vi "CLIENT_read_config_files_to_fgv.vi"(8 "error_in":errorcluster, 11 "all_config_info_in":T1={"main_ini_file"={"SQL Driver"="", "SQL Server"="", "SQL Database"="", "SQL UID"="", "Reference table"="", "Reference history"="", "Archivisation CFG table"="", "Archivisation CFG history"="", "User table"="", "User history"="", "logout timeout [ms]"=0, "records per page"=0, "default language"="", "REF CHG connection IP"="", "REF CHG remote port"=0, "REF CHG local port"=0, "SCANNER COM port"=0, "SCANNER Baud rate"=0, "SCANNER Data bits"=0, "SCANNER Pairity"=enum."None", "SCANNER Stop bits"=10, "SCANNER Flow control"=0, "SCANNER Termination char"=0}, "SQL Password"="", "queue_refnums"={"SQL_EDITOR_queue"=refnum, "SCANNER_queue"=refnum, "SCANNER_data"=refnum, "CLIENT_REF_CHG_queue"=refnum}} {"main_ini_file"."SCANNER Flow control" items=["None"=0, "XON/XOFF"=1, "RTS/CTS"=2, "DTR/DSR"=4]; "main_ini_file"."SCANNER Stop bits" items=["1.0"=10, "1.5"=15, "2.0"=20]}) -> (0 "error_out":errorcluster, 3 "all_config_info_out":T1={"main_ini_file"={"SQL Driver"="", "SQL Server"="", "SQL Database"="", "SQL UID"="", "Reference table"="", "Reference history"="", "Archivisation CFG table"="", "Archivisation CFG history"="", "User table"="", "User history"="", "logout timeout [ms]"=0, "records per page"=0, "default language"="", "REF CHG connection IP"="", "REF CHG remote port"=0, "REF CHG local port"=0, "SCANNER COM port"=0, "SCANNER Baud rate"=0, "SCANNER Data bits"=0, "SCANNER Pairity"=enum."None", "SCANNER Stop bits"=10, "SCANNER Flow control"=0, "SCANNER Termination char"=0}, "SQL Password"="", "queue_refnums"={"SQL_EDITOR_queue"=refnum, "SCANNER_queue"=refnum, "SCANNER_data"=refnum, "CLIENT_REF_CHG_queue"=refnum}} {"main_ini_file"."SCANNER Flow control" items=["None"=0, "XON/XOFF"=1, "RTS/CTS"=2, "DTR/DSR"=4]; "main_ini_file"."SCANNER Stop bits" items=["1.0"=10, "1.5"=15, "2.0"=20]})   [LabVIEW 2019]
uses:
  typedef/CLIENT_all_config_info.ctl
  typedef/CLIENT_main_ini_file.ctl
  queues/typedef/CLIENT_queue_refnums.ctl
  queues/typedef/SQL_EDITOR_queue_element.ctl
  MAIN/SQL_EDITOR/SQL_EDITOR_sequence_state.ctl
  queues/typedef/CLIENT_SCANNER_queue_element.ctl
  MAIN/SCANNER/SCANNER_sequence_state.ctl
  queues/typedef/CLIENT_REF_CHG_queue_element.ctl
  MAIN/reference_changed_connection/CLIENT_REF_CHG_sequence_state.ctl
  FGV/main_ini/FGV_CLIENT_config_info.ctl
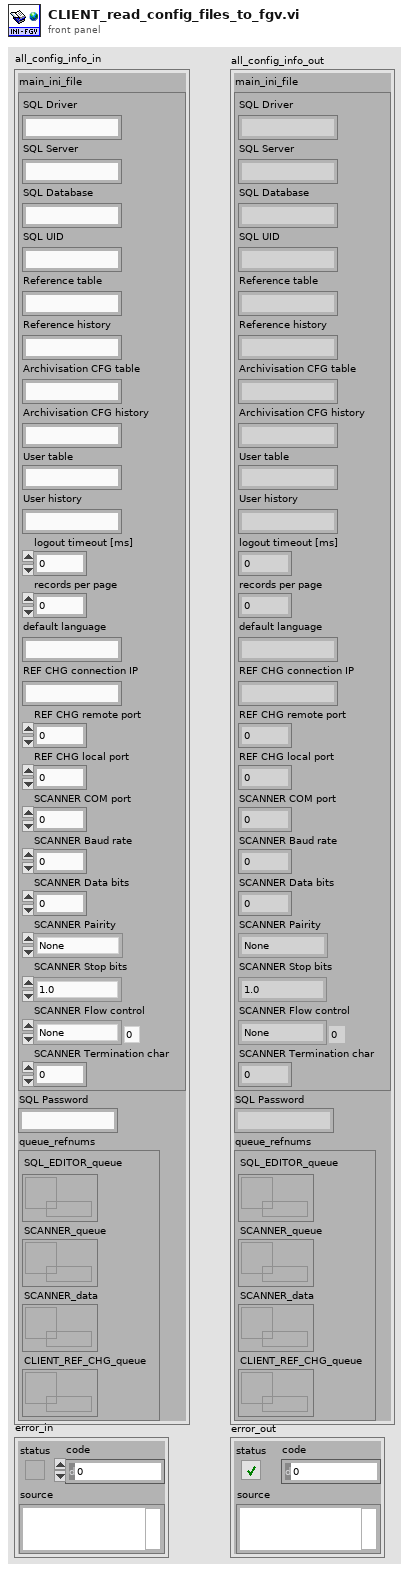
[diagram p1: front panel]
types:
  T1 = typedef "CLIENT_all_config_info.ctl" = cluster{"main_ini_file":T2, "SQL Password":string, "queue_refnums":T3}
  T2 = typedef "CLIENT_main_ini_file.ctl" = cluster{"SQL Driver":string, "SQL Server":string, "SQL Database":string, "SQL UID":string, "Reference table":string, "Reference history":string, "Archivisation CFG table":string, "Archivisation CFG history":string, "User table":string, "User history":string, "logout timeout [ms]":i32, "records per page":i32, "default language":string, "REF CHG connection IP":string, "REF CHG remote port":i32, "REF CHG local port":i32, "SCANNER COM port":u16, "SCANNER Baud rate":u32, "SCANNER Data bits":u16, "SCANNER Pairity":enum16{"None", "Odd", "Even", "Mark", "Space"}, "SCANNER Stop bits":u16, "SCANNER Flow control":u16, "SCANNER Termination char":u8}
  T3 = typedef "CLIENT_queue_refnums.ctl" = cluster{"SQL_EDITOR_queue":refnum<queue>, "SCANNER_queue":refnum<queue>, "SCANNER_data":refnum<queue>, "CLIENT_REF_CHG_queue":refnum<queue>}
  T4 = typedef "FGV_CLIENT_config_info.ctl" = enum16{"initialize", "set", "get"}
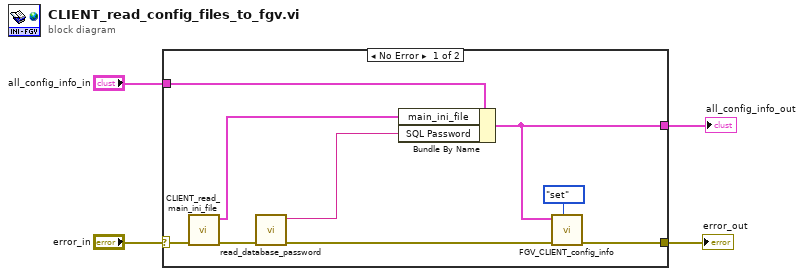
[diagram p0: block diagram]
diagram:
  n1 = case shown="No Error" "error_in" {
    selector: "error_in" -> [w13 w15]
    tunnel: [w11 w15] -> w4
    tunnel: [w5 w14] -> w1
    tunnel: "all_config_info_in" -> [w10 w14]
    frame No Error {
      n2 = call "CLIENT_read_main_ini_file.vi"("error_in"=w13) -> ("error_out"=w9:errorcluster, "main_ini_file_out"=w6:T2)  [unwired: 7 in, 2 out]
      n3 = call "read_database_password.vi"("error_in"=w9) -> ("error_out"=w8:errorcluster, "database_password"=w7:string)  [unwired: 8 in]
      n4 = Bundle By Name(cluster=w10, "main_ini_file"=w6, "SQL Password"=w7) -> (w5:T1)
      n5 = call "FGV_CLIENT_config_info.vi"("options"=FGV_CLIENT_config_info."set", "error_in"=w8, "all_config_info_in"=w5) -> ("error_out"=w11:errorcluster)  [unwired: 7 in, 1 out]
    }
    frame Error {
    }
  }
  "error_out" <- w4
  "all_config_info_out" <- w1
